vi "Get settings chain.vi"(8 "error in (no error)":errorcluster, 11 "RetigaBase in":refnum<class "Retiga.lvclass">) -> (0 "error out":errorcluster, 1 "class name":string[](array[string]), 2 "settings":variant[](array[variant]), 3 "RetigaBase out":refnum<class "Retiga.lvclass">)   [LabVIEW 2012, in "Retiga.lvclass"]
doc: "Returns an array of variants containing the settings clusters of each class in the inheritance chain (lowest child class first), together with an array of all class names in the inheritance chain.\n\nFor classes without settings cluster, the settings chain contains empty variants."
uses:
  Retiga.lvclass
  <vilib>/Distrio/Murmex/Murmex/Murmex.lvclass
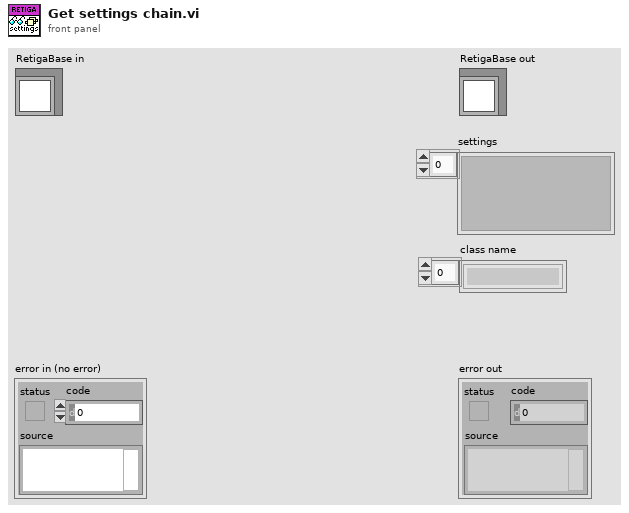
[diagram p1: front panel]
types:
  T1 = typedef "Retiga.lvclass/settings.ctl" = cluster{"Gain":dbl, "Exposure":dbl[unit], "Path":path, "filename":string}
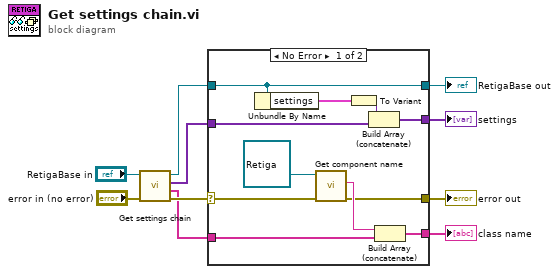
[diagram p0: block diagram]
diagram:
  n1 = call-parent "Get settings chain.vi"("error in (no error)"="error in (no error)", "MurmexBase in"="RetigaBase in") -> ("error out"=w8:errorcluster, "class name"=w6:string[], "settings"=w3:variant[], "MurmexBase out"=w5:refnum<class "Retiga.lvclass">)  [unwired: 6 in]
  n2 = case shown="No Error" w8 {
    selector: w8 -> [w18 w23]
    tunnel: [w16 w23] -> w7
    tunnel: w6 -> [w15 _]
    tunnel: w5 -> [w14 w22]
    tunnel: [w14 w22] -> w4
    tunnel: w3 -> [w13 _]
    tunnel: [w12 _] -> w2
    tunnel: [w11 _] -> w1
    frame No Error {
      n3 = Unbundle By Name(w14) -> ("settings"=w20:T1)
      n4 = call <vilib>:"Get component name.vi"("error in (no error)"=w18, "Murmex in"=refnum<class "Retiga.lvclass"> refnum ("RetigaBase in")) -> ("error out"=w16:errorcluster, "component name"=w19:string)  [unwired: 7 in, 1 out]
      n5 = To Variant(anything=w20) -> (Variant=w21:variant)
      n6 = Build Array (concatenate)(w21, w13) -> (w12:variant[])
      n7 = Build Array (concatenate)(w19, w15) -> (w11:string[])
    }
    frame Error {
    }
  }
  "error out" <- w7
  "RetigaBase out" <- w4
  "settings" <- w2
  "class name" <- w1
